vi "Subscribe.vi"(7 "DataHandler (None)":refnum<class "SubscribedDataHandler.lvclass">, 8 "error in (no error)":errorcluster, 9 "Port":u16, 10 "Address":string, 11 "RemoteDataService in":refnum<class "RemoteDataService.lvclass">) -> (0 "error out":errorcluster, 3 "RemoteDataService out":refnum<class "RemoteDataService.lvclass">)   [LabVIEW 2020, in "Vecto.lvlib" / "RemoteDataService.lvclass"]
uses:
  RemoteDataService.lvclass
  SubscribedDataHandler/SubscribedDataHandler.lvclass
  Subscribe Data.ctl
  Subscription.ctl
  RemoteDataService.lvclass/RemoteDataService.ctl
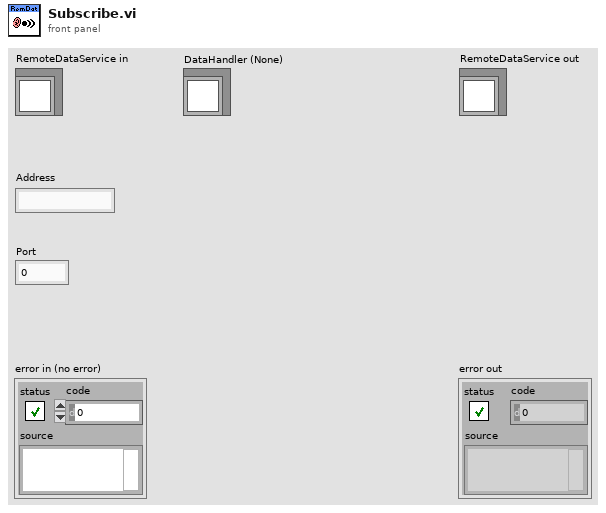
[diagram p1: front panel]
types:
  T1 = typedef "Vecto.lvlib/RemoteDataService.lvclass/Subscribe Data.ctl" = cluster{"Subscription":T2, "DataHandler":refnum<class "SubscribedDataHandler.lvclass">}
  T2 = typedef "Vecto.lvlib/RemoteDataService.lvclass/Subscription.ctl" = cluster{"Multicast Address":string, "Multicast Port":u16}
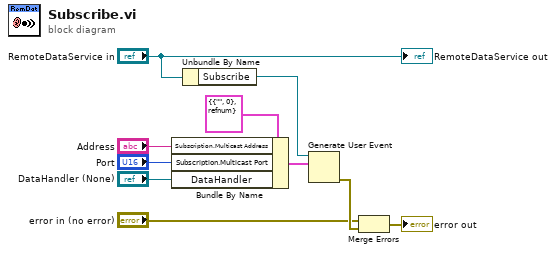
[diagram p0: block diagram]
diagram:
  n1 = Bundle By Name(cluster=T1 {"Subscription"={"Multicast Address"="", "Multicast Port"=0}, "DataHandler"=refnum} ("Subscribe Data"), "Subscription.Multicast Address"="Address", "Subscription.Multicast Port"="Port", "DataHandler"="DataHandler (None)") -> (w6:T1)
  n2 = Unbundle By Name("RemoteDataService in") -> ("Subscribe"=w5:refnum<user-event>)
  n3 = Generate User Event(user event=w5, event data cluster=w6) -> (error out=w4:errorcluster)  [unwired: 2 in, 1 out]
  n4 = Merge Errors("error in (no error)", w4) -> (→"error out":errorcluster)
  "RemoteDataService out" <- "RemoteDataService in"
